vi "FindMaxMin.vi"(0 "x-axis":sgl[](array[numeric]), 1 "y-axis":dbl[](array[numeric])) -> (2 "MaxPosition":dbl format="%#.3p", 3 "MaxValue":dbl format="%#.3f", 4 "MinPosition":dbl format="%#.3f", 5 "MinValue":dbl format="%#.3p")   [LabVIEW 2010]
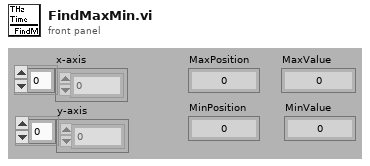
[diagram p1: front panel]
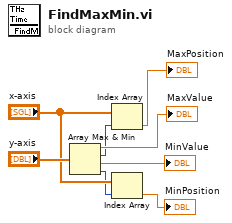
[diagram p0: block diagram]
diagram:
  n1 = Array Max & Min(array="y-axis") -> (max value=→"MaxValue":dbl, max index (indices)=w5:i32, min value=→"MinValue":dbl, min index (indices)=w3:i32)
  n2 = Index Array(array="x-axis", index=w5) -> (element=→"MaxPosition":sgl)
  n3 = Index Array(array="x-axis", index=w3) -> (element=→"MinPosition":sgl)
